vi "Get All Private Data Controls.vi"(8 "error in (no error)":errorcluster, 11 "Class":path) -> (0 "error out":errorcluster, 2 "Private Data Controls":path[](array[path]))   [LabVIEW 2017, in "Composition.lvlib"]
doc: "Returns the paths for all private data clusters in the class hierarchy from most recent to eldest."
uses:
  Composition.lvlib
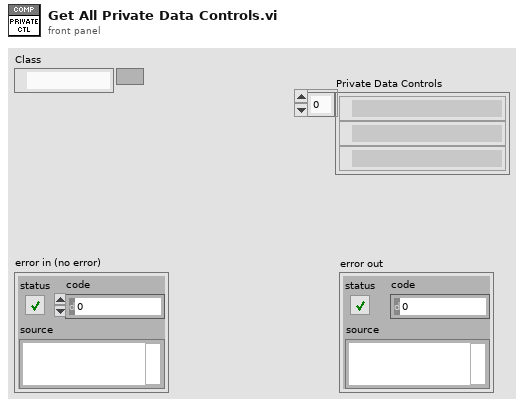
[diagram p1: front panel]
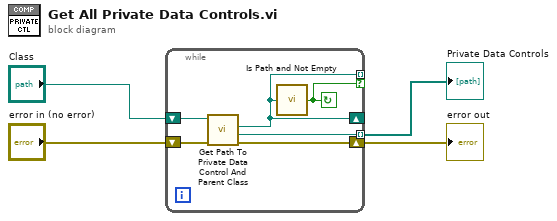
[diagram p0: block diagram]
diagram:
  n1 = while {
    tunnel: [w9] -> w3 mode=indexing
    shift-right: [w6] -> _
    shift-left: "Class" -> [w8]
    shift-right: [w10] -> w4
    shift-left: "error in (no error)" -> [w7]
    tunnel: [w6] -> _ mode=indexing if=w5
    stop <- w5 continue-if-true
    n2 = call "Get Path To Private Data Control And Parent Class.vi"("error in (no error)"=w7, "Class"=w8) -> ("error out"=w10:errorcluster, "Private Data Control"=w9:path, "Parent"=w6:path)  [unwired: 7 in]
    n3 = call <vilib>:"Is Path and Not Empty.vi"("path"=w6) -> ("Is Path and Not Empty?"=w5:bool)  [unwired: 4 in]
  }
  "error out" <- w4
  "Private Data Controls" <- w3
